vi "帧数选择.vi"() -> (5 "AVI Refnum":T2, 6 "初始帧":dbl, 7 "Frame Data":T1, 8 "视频的总帧数":u32, 9 "结束帧":dbl)   [LabVIEW 2018]
uses:
  <vilib>/vision/Avi.llb/IMAQ AVI2 Refnum.ctl
  <vilib>/Utility/error.llb/DialogType.ctl
panel:
  in  "重新选择":bool
  out "结束帧":T3(plugin-control)
  out "初始帧":T3(plugin-control)
  in  "确定按钮":bool
  in  "请输入结束帧":dbl max=241.0
  in  "请输入初始帧":dbl=1.0 min=1.0
  # "帧数选择"
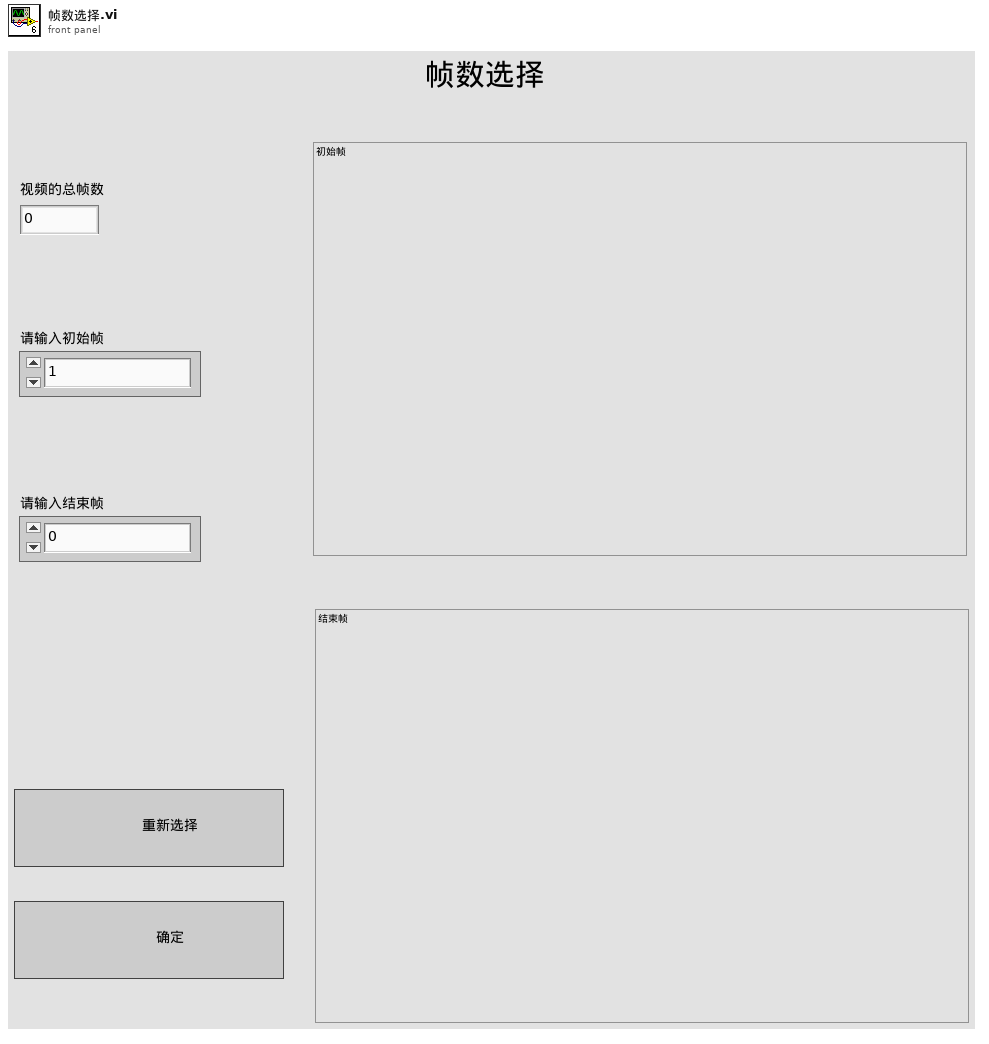
[diagram p1: front panel]
types:
  T1 = cluster{"Width":u32, "Height":u32, "Frames Per Second":u32, "Codec":string, "Has Data":bool}
  T2 = typedef "IMAQ AVI2 Refnum.ctl" = refnum<k20>
  T3 = typedef "IMAQ Image.ctl" = refnum<image>
  T4 = typedef "DialogType.ctl" = u16
  T5 = typedef "Image Type" = u32
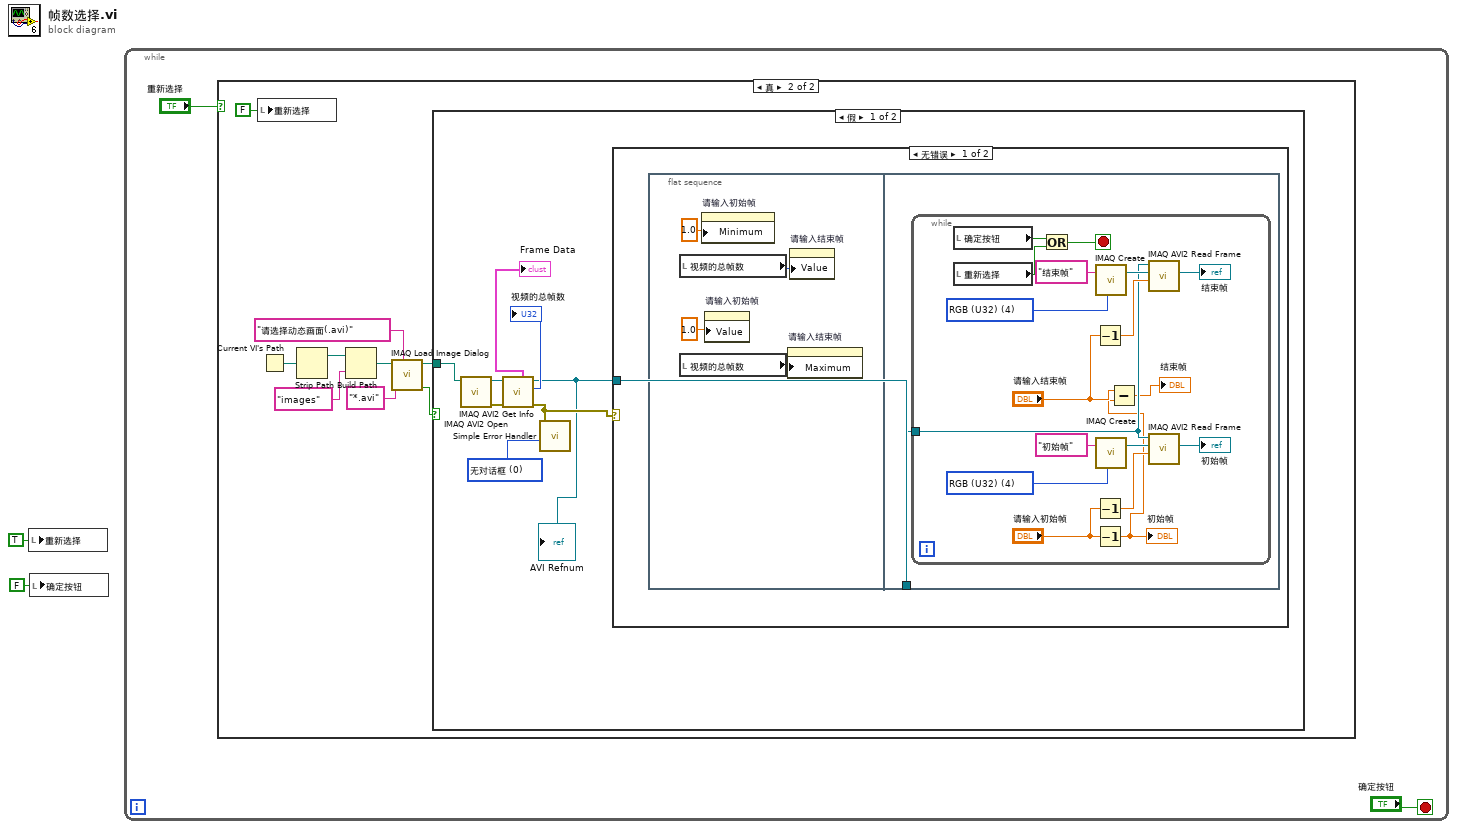
[diagram p0: block diagram]
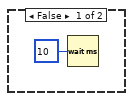
[diagram p2: hidden frame]
diagram:
  n1 = local write "重新选择"(TRUE ("首端按钮")) -> ()
  n2 = local write "确定按钮"(FALSE ("首端按钮")) -> ()
  n3 = while {
    stop <- "确定按钮" stop-if-true
    n4 = case shown="真" "重新选择" {
      frame False {
        n5 = Wait (ms)(milliseconds to wait=u32 10 ("等待时间（毫秒）")) -> ()  [unwired: 1 out]
      }
      frame True {
        n6 = local write "重新选择"(FALSE ("首端按钮")) -> ()
        n7 = Current VI's Path() -> (path=w13:path)
        n8 = Strip Path(path=w13) -> (stripped path=w12:path)  [unwired: 1 out]
        n9 = Build Path(base path=w12, name or relative path="images") -> (appended path=w11:path)
        n10 = call "IMAQ Load Image Dialog"("Prompt"="请选择动态画面(.avi)" ("prompt"), "Pattern"="*.avi", "Start Path"=w11) -> ("Cancelled?"=w6:bool, "Path"=w7:path)  [unwired: 6 in, 1 out]
        n11 = case shown="假" w6 {
          tunnel: w7 -> [w20 _]
          frame False {
            w18 = T4 0 items=["无对话框", "确定信息", "继续或停止信息", "确定信息＋警告", "继续/停止+警告"] ("type of dialog (OK msg:1)")
            n12 = call "IMAQ AVI2 Open"("AVI File Path"=w20) -> ("error out"=w21:errorcluster, "AVI Refnum"=w22:T2)  [unwired: 2 in, 7 out]
            n13 = call "IMAQ AVI2 Get Info"("error in (no error)"=w21, "AVI Refnum"=w22) -> ("error out"=w17:errorcluster, "Number of Frames"=→"视频的总帧数":u32, "AVI Refnum (duplicate)"=w16:T2, "Frame Data"=→"Frame Data":T1)  [unwired: 6 out]
            "AVI Refnum" <- w16
            n14 = call <vilib>:"Simple Error Handler.vi"("type of dialog (OK msg:1)"=w18, "error in (no error)"=w17) -> ()  [unwired: 3 in, 5 out]
            n15 = case shown="无错误" w17 {
              tunnel: w16 -> [w23 _]
              frame No Error {
                n16 = flat-sequence {
                  tunnel: w23 -> [w28]
                  frame #0 {
                    n17 = local read "视频的总帧数"() -> (w27:u32)
                    n18 = local read "视频的总帧数"() -> (w26:u32)
                    n19 = property on="请输入初始帧" class="DigNum (严格)"("Minimum"=1.0 ("数据输入界限:最小值")) -> ()  [unwired: 2 in, 2 out]
                    n20 = property on="请输入初始帧" class="DigNum (严格)"("Value"=1.0 ("数据输入界限:最小值")) -> ()  [unwired: 2 in, 2 out]
                    n21 = property on="请输入结束帧" class="DigNum (严格)"("Maximum"=w26) -> ()  [unwired: 2 in, 2 out]
                    n22 = property on="请输入结束帧" class="DigNum (严格)"("Value"=w27) -> ()  [unwired: 2 in, 2 out]
                  }
                  frame #1 {
                    n23 = while {
                      tunnel: w28 -> [w35]
                      stop <- w32 stop-if-true
                      w38 = T5 4 items=["Grayscale (U8)", "Grayscale (I16)", "Grayscale (SGL)", "Complex (CSG)", "RGB (U32)", "HSL (U32)", "RGB (U64)", "Grayscale (U16)"] ("Image Type")
                      w36 = T5 4 items=["Grayscale (U8)", "Grayscale (I16)", "Grayscale (SGL)", "Complex (CSG)", "RGB (U32)", "HSL (U32)", "RGB (U64)", "Grayscale (U16)"] ("Image Type")
                      n24 = local read "确定按钮"() -> (w34:bool)
                      n25 = local read "重新选择"() -> (w33:bool)
                      n26 = Or(x=w34, y=w33) -> (x .or. y?=w32:bool)
                      n27 = Decrement(x="请输入结束帧") -> (x-1=w41:dbl)
                      n28 = Decrement(x="请输入初始帧") -> (x-1=w40:dbl)
                      n29 = Decrement(x="请输入初始帧") -> (x-1=w30:dbl)
                      "初始帧" <- w30
                      n30 = call "IMAQ Create"("Image Name"="结束帧", "Image Type"=w38) -> ("New Image"=w42:T3)  [unwired: 2 in, 2 out]
                      n31 = call "IMAQ Create"("Image Name"="初始帧", "Image Type"=w36) -> ("New Image"=w43:T3)  [unwired: 2 in, 2 out]
                      n32 = Subtract(x="请输入结束帧", y=w30) -> (x-y=→"结束帧":dbl)
                      n33 = call "IMAQ AVI2 Read Frame"("Frame Number"=w41, "Image"=w42, "AVI Refnum"=w35) -> ("Image Out"=→"结束帧":T3)  [unwired: 1 in, 7 out]
                      n34 = call "IMAQ AVI2 Read Frame"("Frame Number"=w40, "Image"=w43, "AVI Refnum"=w35) -> ("Image Out"=→"初始帧":T3)  [unwired: 1 in, 7 out]
                    }
                  }
                }
              }
              frame Error {
              }
            }
          }
          frame True {
          }
        }
      }
    }
  }
